vi "Chirplet TDR.vi"() -> ()   [LabVIEW 2023]
doc: "This example shows the application of the Time Frequency Analysis VIs in Time Domain Reflectometry (TDR). \n\nA TDR is an instrument that characterizes and locates faults in cables. You can transmit a chirplet along a cable and receive the reflected signal. The reflected signal also is a chirplet but has different time center, amplitude, and others. You can characterize and locate faults in the cable based on the difference between the transmitted chirplet and the reflected chirplet. \n\nA TDR signal contains both the transmitted and the reflected chirplets. One of the challenges in the applications of TDR is how to separate and extract parameters of the transmitted and the reflected chirplets. This example simulates the TDR signal from a cable and uses the TFA Adaptive Transform VI to extract the parameters of these two chirplets. \n\n<b>Instructions:</b>\n1) Run this VI.\n2) Specify the cable parameters in the <b>Parameters of Cable</b> section to simulate a TDR signal.\n3) Observe the measured parameters."
uses:
  <vilib>/addons/Time Frequency Analysis/Transform.llb/TFA Adaptive Transform (Waveform).vi
  <vilib>/addons/_Advanced Signal Processing/NI_AdvSigProcTFA.lvlib
panel:
  in  "Stop":bool
  out "Reflectance":dbl=0.431278352121774
  in  "test parameters":T1={"Sample Rate [Hz]"=1000000.0, "Max Length [m]"=1.0, "SNR [dB]"=26.0} {"SNR [dB]" format="%.2f"; "Max Length [m]" format="%.2f"; "Sample Rate [Hz]" format="%.2p"}
  in  "Refletion":T2={"Reflectance "=0.5, "Phase shift (deg)"=-63.20559286450312} {"Reflectance" format="%.2f"}
  in  "Cable":T3={"Length (m) "=0.43125, "Attenuation (dB/m)"=20.0, "Propagation speed (m/s)"=1500.0} {"Propagation speed (m/s)" format="%.2f"; "Attenuation (dB/m)" format="%.2f"; "Length (m)" format="%.4f"}
  in  "source chirplet":T4={"F Central [Hz]"=50000.0, "Bandwidth [Hz]"=50000.0, "Chirplet Length [m]"=0.2, "Amplitude [EU]"=10.0} {"Amplitude [EU]" format="%.2f"; "Chirplet Length [m]" format="%.4f"; "Bandwidth [Hz]" format="%.2p"; "F Central [Hz]" format="%.2p"}
  out "Phase (deg)":dbl=-63.25423590904824
  out "Length (m)":dbl=0.431278352121774
  out "Simulated TDR Signal":waveform(dbl)(graph)
  # "Overview: Shows the application of the Time Frequency Analysis VIs in Time Domain Reflectometry (TDR).\nRequirements: LabVIEW Full Development System, Advanced Signal Processing Toolkit\nInstructions: \n1. Run this VI.\n2. Specify the cable parameters in the Parameters of Cable section to simulate a TDR signal.\n3. Observe the measured parameters.\n4. Click Stop to stop the VI."
  # "Parameters of Cable"
  # "Measured Parameters of the Cable"
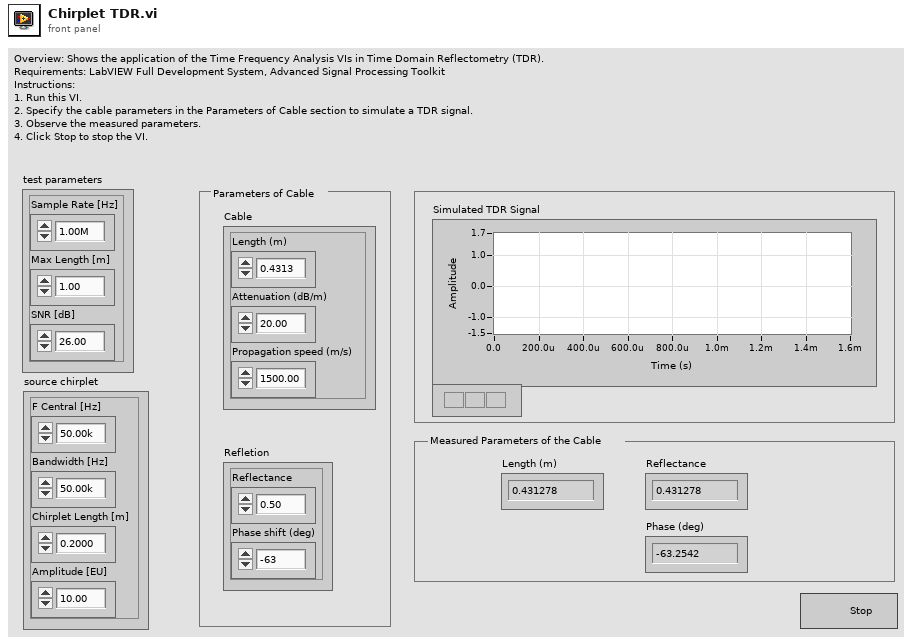
[diagram p1: front panel]
types:
  T1 = cluster{"Sample Rate [Hz]":dbl, "Max Length [m]":dbl, "SNR [dB]":dbl}
  T2 = cluster{"Reflectance ":dbl, "Phase shift (deg)":dbl}
  T3 = cluster{"Length (m) ":dbl, "Attenuation (dB/m)":dbl, "Propagation speed (m/s)":dbl}
  T4 = cluster{"F Central [Hz]":dbl, "Bandwidth [Hz]":dbl, "Chirplet Length [m]":dbl, "Amplitude [EU]":dbl}
  T5 = cluster{"amplitude":cdb, "standard deviation":dbl, "center":dbl, "frequency":dbl, "chirp rate":dbl}[]
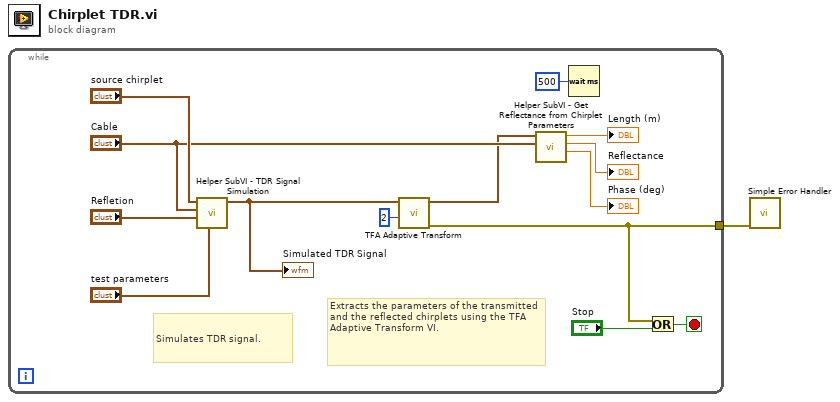
[diagram p0: block diagram]
diagram:
  n1 = while {
    tunnel: [w2] -> w1
    stop <- w4 stop-if-true
    # "Simulates TDR signal."
    # "Extracts the parameters of the transmitted and the reflected chirplets using the TFA Adaptive Transform VI."
    n2 = call "Helper SubVI - TDR Signal Simulation.vi"("test parameters"="test parameters", "target parameters"="Refletion", "path parameters"="Cable", "source chirplet"="source chirplet") -> ("time waveform"=w14:waveform(dbl))  [unwired: 7 out]
    "Simulated TDR Signal" <- w14
    n3 = call-poly <vilib>:"TFA Adaptive Transform.vi"("number of terms"=2, "signal"=w14) -> ("error out"=w2:errorcluster, "chirplet info"=w6:T5)  [unwired: 1 in, 7 out]
    n4 = call "Helper SubVI - Get Reflectance from Chirplet Parameters.vi"("media parameters"="Cable", "ADT paras"=w6) -> ("Phase [Deg]"=→"Phase (deg)":dbl, "Reflectance"=→"Reflectance":dbl, "Length [m]"=→"Length (m)":dbl)  [unwired: 1 in, 6 out]
    n5 = Wait (ms)(milliseconds to wait=u32 500 ("millisecond multiple")) -> ()  [unwired: 1 out]
    n6 = Or(x=w2, y="Stop") -> (x .or. y?=w4:bool)
  }
  n7 = call <vilib>:"Simple Error Handler.vi"("error in (no error)"=w1) -> ()  [unwired: 1 in, 8 out]
